vi "Stop Core.vi"(10 "final error code":i32, 11 "Device in":refnum<class "Device.lvclass">) -> (3 "Device out":refnum<class "Device.lvclass">)   [LabVIEW 2015, in "DAQ Device.lvlib" / "Device.lvclass"]
doc: "(<B>Filename</B>: Actor Framework.lvlib:Actor.lvclass:Stop Core.vi)\n\nDefines what the actor does before it stops. Use the <B>final error code</B> input to determine whether the actor shut down in response to an error.\n\nBy default, this method does nothing. A descendant class may override it to define behavior, such as shutting down any processes the actor initiated in its override of the Actor Core method."
uses:
  Device.lvclass
  <vilib>/MSR Consulting, LLC/General Reuse/SuperActor/SuperActor.lvclass/SuperActor.ctl
  Device.lvclass/Device.ctl
  <vilib>/MSR Consulting, LLC/General Reuse/SuperActor/Read Log Session.vi
  <vilib>/MSR Consulting, LLC/General Reuse/SuperActor/Read ID.vi
  <vilib>/MSR Consulting, LLC/General Reuse/Session APIs/_Session Fwk/Session - Root.lvclass
  <vilib>/MSR Consulting, LLC/Configurable Device/Configurable Device.lvclass
  <vilib>/MSR Consulting, LLC/General Reuse/SuperActor/SuperActor.lvclass
  <vilib>/MSR Consulting, LLC/General Reuse/Session APIs/Session Log/System Log.lvclass
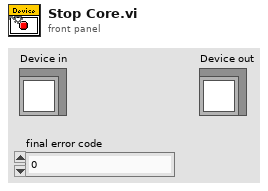
[diagram p1: front panel]
types:
  T1 = typedef "Session - Root.lvclass/Session Handle.ctl" = refnum<data-value>
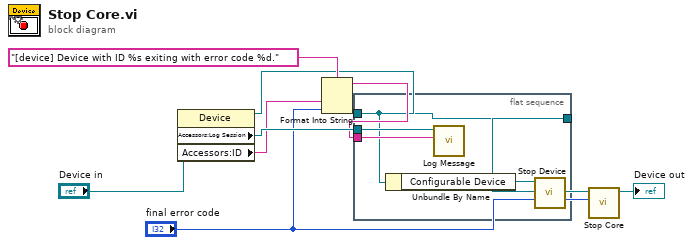
[diagram p0: block diagram]
diagram:
  n1 = property class="Device"(reference="Device in") -> (reference out=w2:refnum<class "Device.lvclass">, "Accessors:Log Session"=w7:T1, "Accessors:ID"=w4:string)  [unwired: 1 in, 1 out]
  n2 = Format Into String(format string="[device] Device with ID %s exiting with error code %d.", w4, "final error code") -> (resulting string=w3:string)  [unwired: 2 in, 1 out]
  n3 = flat-sequence {
    tunnel: w7 -> [w13]
    tunnel: w3 -> [w12]
    tunnel: w2 -> [w10]
    tunnel: [w10] -> w1
    frame #0 {
      n4 = Unbundle By Name(w10) -> ("Configurable Device"=w11:refnum<class "Configurable Device.lvclass">)
      n5 = call <vilib>:"Log Message.vi"("MSG In"=w12, "session in"=w13) -> ()  [unwired: 8 in, 2 out]
      n6 = call-dynamic "Stop Device.vi"("Configurable Device in"=w11) -> ()  [unwired: 9 in, 2 out]
    }
  }
  n7 = call-parent "Stop Core.vi"("final error code"="final error code", "Ex Nested in"=w1) -> ("Ex Nested out"=→"Device out":refnum<class "Device.lvclass">)  [unwired: 9 in]
